vi "제목없음 1 (SubVI).vi"(9 "문자열 입력":string, 10 "불리언":bool, 11 "문자열 3":string) -> (3 "문자열 출력":string)   [LabVIEW 2018]
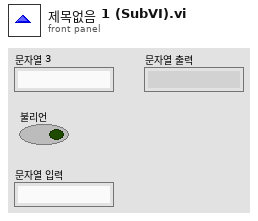
[diagram p1: front panel]
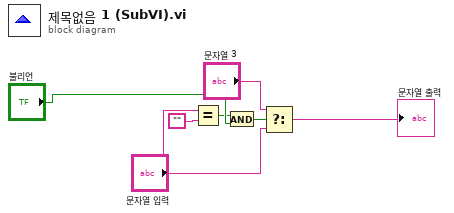
[diagram p0: block diagram]
diagram:
  n1 = Equal?(x="문자열 입력", y="") -> (x = y?=w1:bool)
  n2 = And(x=w1, y="불리언") -> (x .and. y?=w3:bool)
  n3 = Select(t="문자열 3", s=w3, f="문자열 입력") -> (s? t:f=→"문자열 출력":string)
